vi "Error.vi"(8 "error in (no error)":errorcluster, 10 "Variant":variant) -> (0 "error out":errorcluster)   [LabVIEW 2018, in "Module Template.lvlib"]
doc: "Send Error Message to the Queue."
uses:
  Private Controls/Message Cluster.ctl
  Private Controls/Message enum.ctl
  Module Template.lvlib
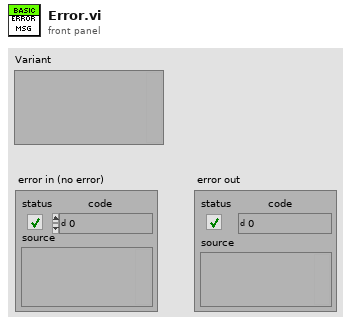
[diagram p1: front panel]
types:
  T1 = typedef "Module Template.lvlib/Message Cluster.ctl" = cluster{"Message":T2, "Data":variant}
  T2 = typedef "Module Template.lvlib/Message enum.ctl" = enum16{"Initialize", "Error", "Exit"}
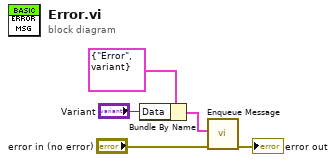
[diagram p0: block diagram]
diagram:
  n1 = Bundle By Name(cluster=T1 {"Message"=enum."Error", "Data"=variant} ("Message Cluster"), "Data"="Variant") -> (w1:T1)
  n2 = call "Enqueue Message.vi"("error in (no error)"="error in (no error)", "Element"=w1) -> ("error out"=→"error out":errorcluster)  [unwired: 9 in]
